vi "PixelatedDetectorP0.vi"() -> ()   [LabVIEW 2018]
panel:
  out "Intensity Graph":dbl[][](graph)
  out "XY Graph":cluster{dbl[], dbl[]}(graph)
  in  "eField":dbl
  in  "height":dbl
  in  "bField":dbl
  in  "velocity":dbl
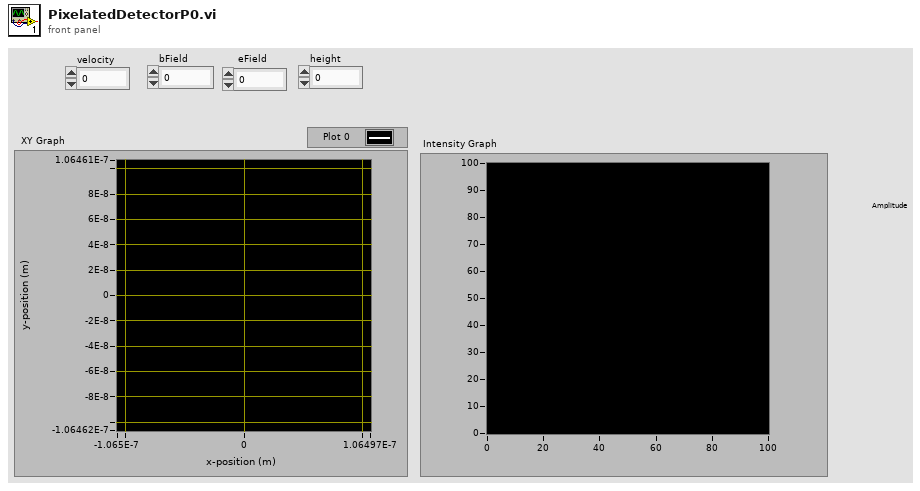
[diagram p1: front panel]
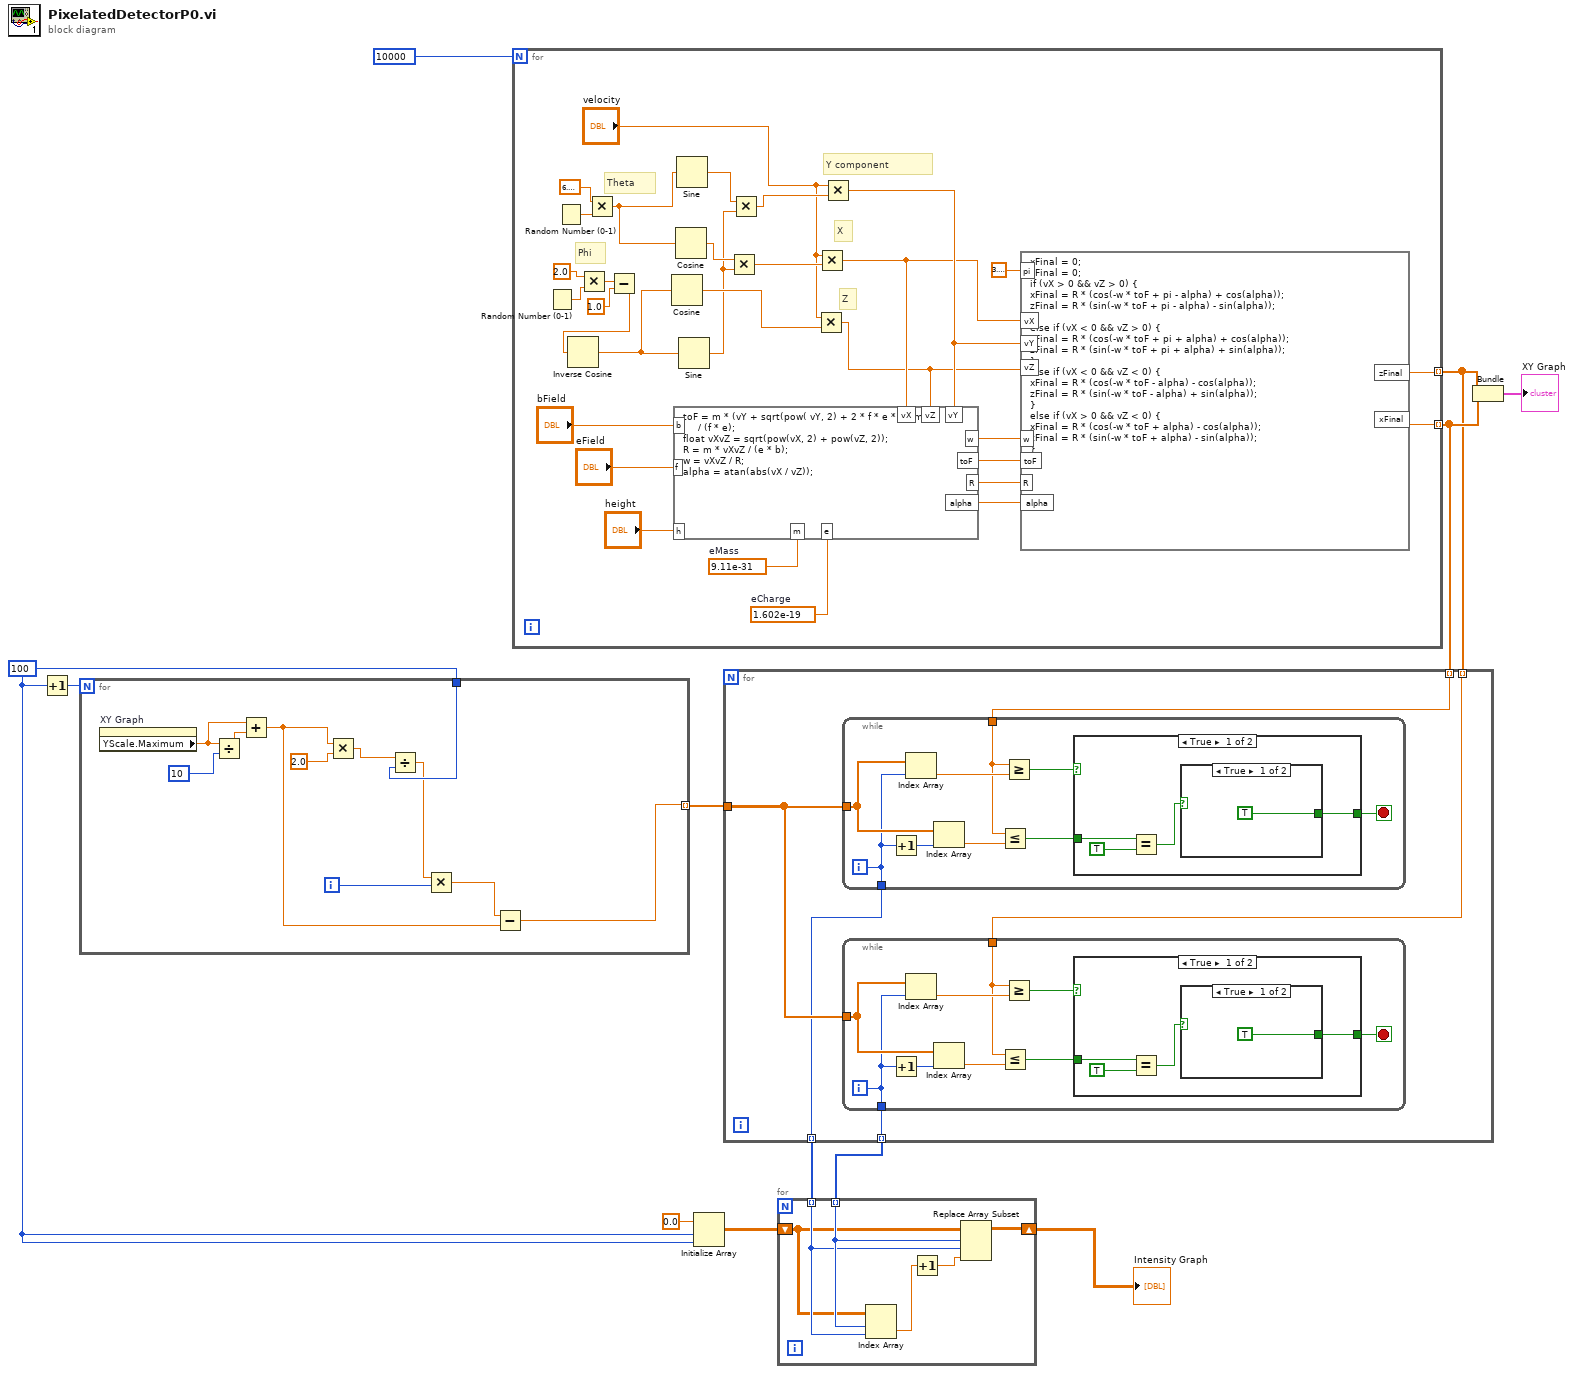
[diagram p0: block diagram]
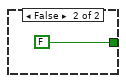
[diagram p2: hidden frame]
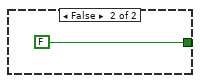
[diagram p3: hidden frame]
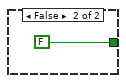
[diagram p4: hidden frame]
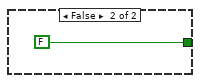
[diagram p5: hidden frame]
diagram:
  w5 = 100
  n1 = Increment(x=w5) -> (x+1=w11:i32)
  n2 = for {
    N: w11 -> [_]
    tunnel: [w23] -> w6 mode=indexing
    tunnel: w5 -> [w20]
    i -> [w19]
    n3 = property on="XY Graph" class="XYGraph (strict)"() -> ("YScale.Maximum"=w14:dbl)  [unwired: 2 in, 2 out]
    n4 = Divide(x=w14, y=10) -> (x/y=w15:dbl)
    n5 = Add(x=w14, y=w15) -> (x+y=w13:dbl)
    n6 = Multiply(x=w13, y=2.0) -> (x*y=w21:dbl)
    n7 = Divide(x=w21, y=w20) -> (x/y=w18:dbl)
    n8 = Multiply(x=w18, y=w19) -> (x*y=w17:dbl)
    n9 = Subtract(x=w17, y=w13) -> (x-y=w23:dbl)
  }
  n10 = for {
    N: 10000 -> [_]
    tunnel: [w32] -> w9 mode=indexing
    tunnel: [w31] -> w10 mode=indexing
    w25 = 9.11e-31  # eMass
    w26 = 1.602e-19  # eCharge
    # "Phi"
    # "Theta"
    # "Z"
    # "X"
    # "Y component"
    n11 = Random Number (0-1)() -> (number: 0 to 1=w49:dbl)
    n12 = Random Number (0-1)() -> (number: 0 to 1=w52:dbl)
    n13 = Multiply(x=2.0, y=w49) -> (x*y=w48:dbl)
    n14 = Multiply(x=6.283185307179586, y=w52) -> (x*y=w46:dbl)
    n15 = Subtract(x=w48, y=1.0) -> (x-y=w45:dbl)
    n16 = Inverse Cosine(1:w45) -> (0:w44:dbl)
    n17 = Cosine(x=w44) -> (cos(x)=w43:dbl)
    n18 = Cosine(x=w46) -> (cos(x)=w40:dbl)
    n19 = Sine(x=w46) -> (sin(x)=w42:dbl)
    n20 = Sine(x=w44) -> (sin(x)=w39:dbl)
    n21 = Multiply(x=w40, y=w39) -> (x*y=w38:dbl)
    n22 = Multiply(x=w42, y=w39) -> (x*y=w41:dbl)
    n23 = Multiply(x="velocity", y=w43) -> (x*y=w35:dbl)
    n24 = Multiply(x="velocity", y=w38) -> (x*y=w36:dbl)
    n25 = Multiply(x="velocity", y=w41) -> (x*y=w37:dbl)
    n26 = formula code="toF = m * (vY + sqrt(pow( vY, 2) + 2 * f * e * h / m))\n     / (f * e);\nfloat vXvZ = sqrt(pow(vX, 2) + pow(vZ, 2));\nR = m * vXvZ / (e * b);\nw = vXvZ / R;\nalpha = atan(abs(vX / vZ));"("f"="eField", "h"="height", "vY"=w37, "m"=w25, "e"=w26, "vX"=w36, "vZ"=w35, "b"="bField") -> ("toF"=w53:dbl, "w"=w34:dbl, "R"=w29:dbl, "alpha"=w33:dbl)
    n27 = formula code="xFinal = 0;\nzFinal = 0;\nif (vX > 0 && vZ > 0) {\nxFinal = R * (cos(-w * toF + pi - alpha) + cos(alpha));\nzFinal = R * (sin(-w * toF + pi - alpha) - sin(alpha));\n}\nelse if (vX < 0 && vZ > 0) {\nxFinal = R * (cos(-w * toF + pi + alpha) + cos(alpha));\nzFinal = R * (sin(-w * toF + pi + alpha) + sin(alpha));\n}\nelse if (vX < 0 && vZ < 0) {\nxFinal = R * (cos(-w * toF - alpha) - cos(alpha));\nzFinal = R * (sin(-w * toF - alpha) + sin(alpha));\n}\nelse if (vX > 0 && vZ < 0) {\nxFinal = R * (cos(-w * toF + alpha) - cos(alpha));\nzFinal = R * (sin(-w * toF + alpha) - sin(alpha));\n}"("vY"=w37, "toF"=w53, "vX"=w36, "vZ"=w35, "w"=w34, "R"=w29, "alpha"=w33, "pi"=3.141592653589793) -> ("zFinal"=w32:dbl, "xFinal"=w31:dbl)
  }
  n28 = Initialize Array(0.0, w5, w5) -> (w4:dbl[][])
  n29 = for {
    tunnel: w10 -> [w59] mode=indexing
    tunnel: w9 -> [w58] mode=indexing
    tunnel: w6 -> [w57]
    tunnel: [w56] -> w3 mode=indexing
    tunnel: [w55] -> w2 mode=indexing
    n30 = while {
      tunnel: w57 -> [w84]
      tunnel: w59 -> [w81]
      tunnel: [w78] -> w56
      i -> [w78]
      stop <- w77 stop-if-true
      n31 = Increment(x=w78) -> (x+1=w83:i32)
      n32 = Index Array(array=w84, index=w78) -> (element=w82:dbl)
      n33 = Index Array(array=w84, index=w83) -> (element=w80:dbl)
      n34 = Less Or Equal?(x=w81, y=w80) -> (x <= y?=w79:bool)
      n35 = Greater Or Equal?(x=w81, y=w82) -> (x >= y?=w76:bool)
      n36 = case shown="True" w76 {
        tunnel: w79 -> [w87 _]
        tunnel: [w85 FALSE] -> w77
        frame True {
          n37 = Equal?(x=w87, y=TRUE) -> (x = y?=w86:bool)
          n38 = case shown="True" w86 {
            tunnel: [TRUE FALSE] -> w85
            frame True {
            }
            frame False {
            }
          }
        }
        frame False {
        }
      }
    }
    n39 = while {
      tunnel: w57 -> [w68]
      tunnel: w58 -> [w65]
      tunnel: [w62] -> w55
      i -> [w62]
      stop <- w61 stop-if-true
      n40 = Increment(x=w62) -> (x+1=w67:i32)
      n41 = Index Array(array=w68, index=w62) -> (element=w66:dbl)
      n42 = Index Array(array=w68, index=w67) -> (element=w64:dbl)
      n43 = Less Or Equal?(x=w65, y=w64) -> (x <= y?=w63:bool)
      n44 = Greater Or Equal?(x=w65, y=w66) -> (x >= y?=w60:bool)
      n45 = case shown="True" w60 {
        tunnel: w63 -> [w71 _]
        tunnel: [w69 FALSE] -> w61
        frame True {
          n46 = Equal?(x=w71, y=TRUE) -> (x = y?=w70:bool)
          n47 = case shown="True" w70 {
            tunnel: [TRUE FALSE] -> w69
            frame True {
            }
            frame False {
            }
          }
        }
        frame False {
        }
      }
    }
  }
  n48 = for {
    tunnel: w2 -> [w97] mode=indexing
    tunnel: w3 -> [w96] mode=indexing
    shift-right: [w92] -> w1
    shift-left: w4 -> [w93]
    n49 = Index Array(array=w93, index (row)=w97, index (col)=w96) -> (element=w94:dbl)
    n50 = Increment(x=w94) -> (x+1=w95:dbl)
    n51 = Replace Array Subset(array=w93, new element=w95, index (row)=w97, index (col)=w96) -> (w92:dbl[][])
  }
  "Intensity Graph" <- w1
  n52 = Bundle(w9, w10) -> (→"XY Graph":cluster{dbl[], dbl[]})  [unwired: 1 in]
